vi "Add Weighted Images (Greyscale).vi"(5 "B":dbl=0.5, 6 "C (Default: 0)":dbl, 7 "A":dbl=0.5, 8 "error in (no error)":errorcluster, 9 "Greyscale Destination in":T1, 10 "Greyscale Image B in":T1, 11 "Greyscale Image A in":T1) -> (0 "error out":errorcluster, 3 "Greyscale Destination":T1)   [LabVIEW 2020, in "image.lvlib"]
doc: "Combine two images A and B scaled by their corresponding scaling factors - with the addition of an optional constant. Pixel values will saturate at their maximum values."
uses:
  image.lvlib
  Greyscale Image.ctl
  2e5e2c88-b721-4a80-abe1-d690325a547c.vi
  <vilib>/Utility/error.llb/Error Cluster From Error Code.vi
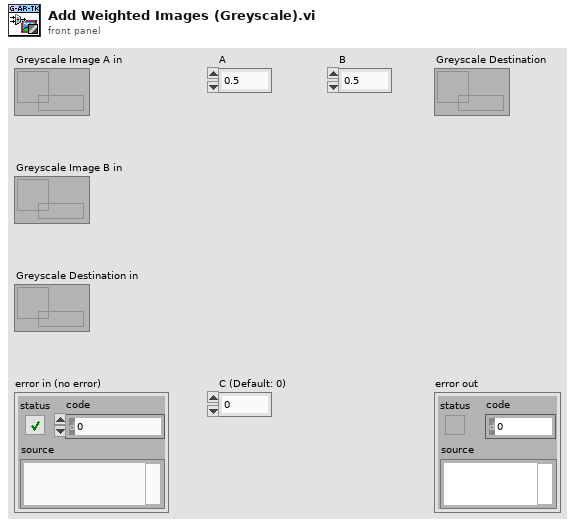
[diagram p1: front panel]
types:
  T1 = typedef "image.lvlib/Greyscale Image.ctl" = refnum<data-value>
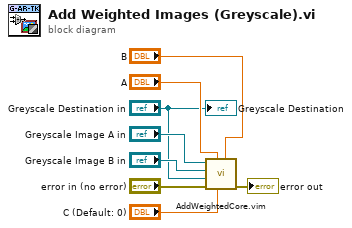
[diagram p0: block diagram]
diagram:
  n1 = call "AddWeightedCore.vim"("B"="B", "C"="C (Default: 0)", "A"="A", "error in (no error)"="error in (no error)", "Dst"="Greyscale Destination in", "Image B"="Greyscale Image B in", "Image A"="Greyscale Image A in") -> ("error out"=→"error out":errorcluster)  [unwired: 4 in]
  "Greyscale Destination" <- "Greyscale Destination in"
